vi "_UpdateRange.vi"(11 "Array":refnum<vi>[](array[refnum])) -> ()   [LabVIEW 2017, in "XTriPhaseGraph.xctl"]
uses:
  XTriPhaseGraph.xctl
  <vilib>/Utility/miscctls.llb/LVRangeTypeDef.ctl
panel:
  out "Array 4":string[](array[string])
  out "Array 3":T1[](array[typedef])
  out "Array 2":T1[](array[typedef])
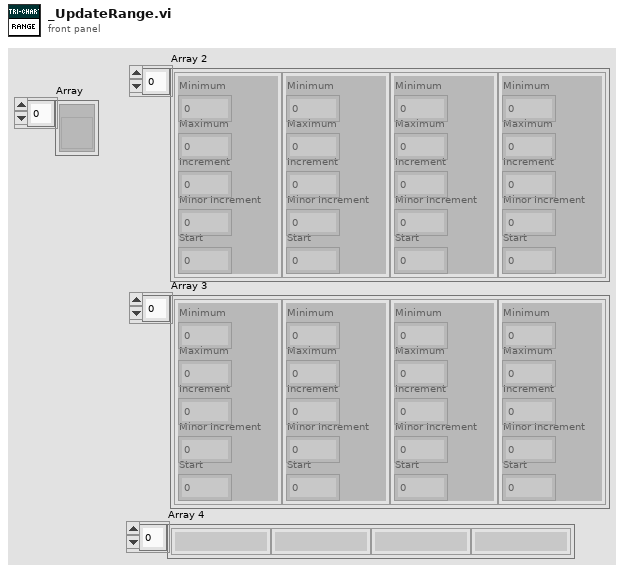
[diagram p1: front panel]
types:
  T1 = typedef "LVRangeTypeDef.ctl" = cluster{"Minimum":dbl, "Maximum":dbl, "Increment":dbl, "Minor Increment":dbl, "Start":dbl}
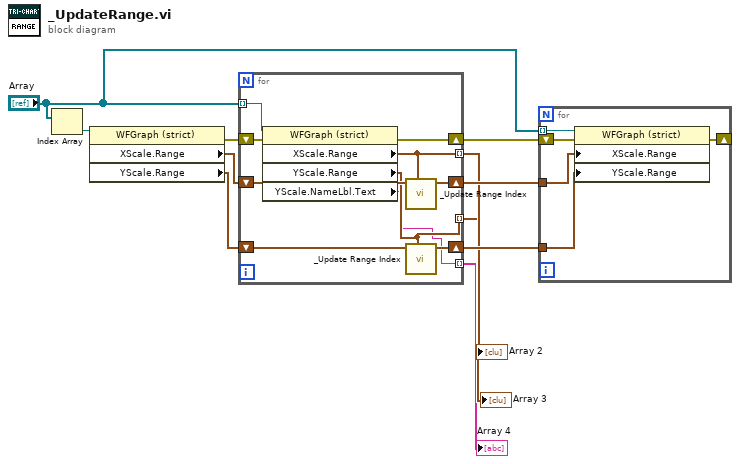
[diagram p0: block diagram]
diagram:
  n1 = Index Array(array="Array") -> (element=w9:refnum<vi>)  [unwired: 1 in]
  n2 = property class="WFGraph (strict)"(reference=w9) -> (error out=w10:errorcluster, "XScale.Range"=w8:T1, "YScale.Range"=w7:T1)  [unwired: 1 in, 1 out]
  n3 = for {
    shift-right: [w21] -> w11
    shift-left: w10 -> [w20]
    tunnel: "Array" -> [w19] mode=indexing
    shift-right: [w18] -> w5
    shift-left: w8 -> [w17]
    shift-right: [w15] -> w6
    shift-left: w7 -> [w16]
    tunnel: [w14] -> w4 mode=indexing
    tunnel: [w13] -> w3 mode=indexing
    tunnel: [w12] -> w1 mode=indexing
    n4 = property class="WFGraph (strict)"(reference=w19, error in=w20) -> (error out=w21:errorcluster, "XScale.Range"=w14:T1, "YScale.Range"=w13:T1, "YScale.NameLbl.Text"=w12:string)  [unwired: 1 out]
    n5 = call "_Update Range Index.vi"("Refrence"=w14, "XScale.Range in"=w17) -> ("XScale.Range out"=w18:T1)  [unwired: 9 in]
    n6 = call "_Update Range Index.vi"("Refrence"=w13, "XScale.Range in"=w16) -> ("XScale.Range out"=w15:T1)  [unwired: 9 in]
  }
  "Array 2" <- w4
  "Array 3" <- w3
  "Array 4" <- w1
  n7 = for {
    tunnel: w5 -> [w25]
    tunnel: w6 -> [w24]
    tunnel: "Array" -> [w23] mode=indexing
    shift-right: [w22] -> _
    shift-left: w11 -> [w26]
    n8 = property class="WFGraph (strict)"(reference=w23, error in=w26, "XScale.Range"=w25, "YScale.Range"=w24) -> (error out=w22:errorcluster)  [unwired: 1 out]
  }
